vi "Init_Instr.vi"(8 "error in (no error)":errorcluster caption="entrée d'erreur (pas d'erreur)", 11 "Class Instrument Multimeter en entrée":refnum<class "Class Instrument LED_Analyser.lvclass">) -> (0 "error out":errorcluster caption="sortie d'erreur", 3 "Class Instrument Multimeter en sortie":refnum<class "Class Instrument LED_Analyser.lvclass">)   [LabVIEW 2020, in "Library Instrument & Equipement.lvlib" / "Library Instruments.lvlib" / "Class Instrument LED_Analyser.lvclass"]
uses:
  Class Instrument LED_Analyser.lvclass
  Class Instrument LED_Analyser.lvclass/Class Instrument LED_Analyser.ctl
  Instrument (Default)/Class Instrument (Default).lvclass
  LED Analyser/Class Led Analyser (Default)/Class LED Analyser (Default).lvclass
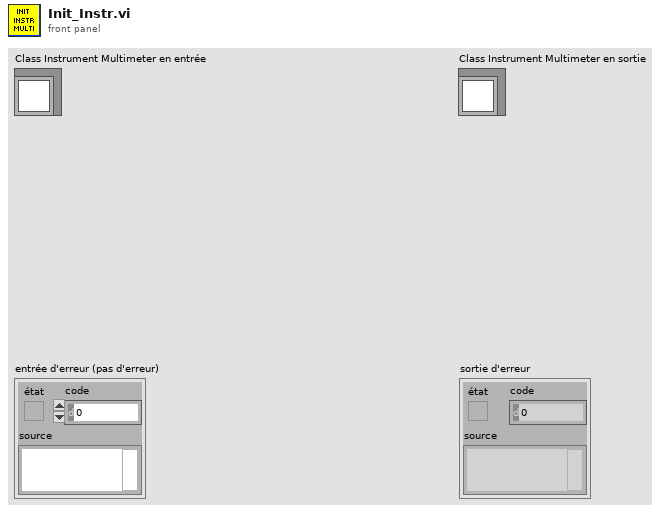
[diagram p1: front panel]
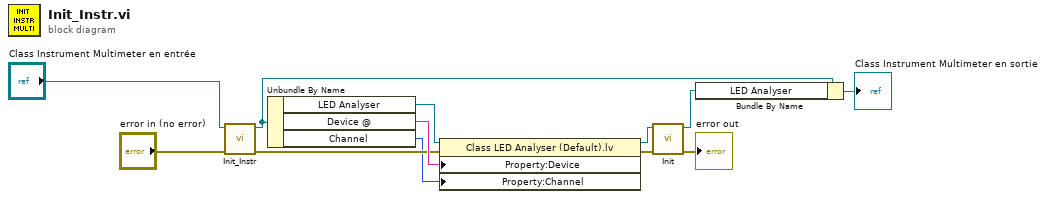
[diagram p0: block diagram]
diagram:
  n1 = call-parent "Init_Instr.vi"("error in (no error)"="error in (no error)", "Class Instrument (Default) en entrée"="Class Instrument Multimeter en entrée") -> ("error out"=w8:errorcluster, "Class Instrument (Default) en sortie"=w6:refnum<class "Class Instrument LED_Analyser.lvclass">)  [unwired: 8 in]
  n2 = Unbundle By Name(w6) -> ("LED Analyser"=w10:refnum<class "Class LED Analyser (Default).lvclass">, "Device @"=w9:string, "Channel"=w1:u16)
  n3 = property class="Class LED Analyser (Default).lv"(reference=w10, error in=w8, "Property:Device"=w9, "Property:Channel"=w1) -> (reference out=w3:refnum<class "Class LED Analyser (Default).lvclass">, error out=w5:errorcluster)
  n4 = call-dynamic "Init.vi"("error in (no error)"=w5, "Class LED Analyser in"=w3) -> ("error out"=→"error out":errorcluster, "Class LED Analyser Out"=w2:refnum<class "Class LED Analyser (Default).lvclass">)  [unwired: 8 in]
  n5 = Bundle By Name(cluster=w6, "LED Analyser"=w2) -> (→"Class Instrument Multimeter en sortie":refnum<class "Class Instrument LED_Analyser.lvclass">)
